vi "MFL_Check_Queue.vi"(0 "queue":refnum<queue>, 2 "error in (no error)":errorcluster) -> (3 "MFL_Monitor":T1 {"Osc 3 Freq" min=0.0 max=510000.0 format="%#_11g"; "Osc 2 Freq" min=0.0 max=510000.0 format="%#_11g"; "Osc 1 Freq" min=0.0 max=510000.0 format="%#_11g"; "Osc 0 Freq" min=0.0 max=510000.0 format="%#_11g"; "Demod Sample out 3"."Aux In 1 (V)" format="%#_5p"; "Demod Sample out 3"."Aux In 0 (V)" format="%#_5p"; "Demod Sample out 3"."X (Vrms)" format="%#_5p"; "Demod Sample out 3"."Y (Vrms)" format="%#_5p"; "Demod Sample out 3"."Osc Phase (rad)" format="%#.3g"; "Demod Sample out 2"."Aux In 1 (V)" format="%#_5p"; "Demod Sample out 2"."Aux In 0 (V)" format="%#_5p"; "Demod Sample out 2"."X (Vrms)" format="%#_5p"; "Demod Sample out 2"."Y (Vrms)" format="%#_5p"; "Demod Sample out 2"."Osc Phase (rad)" format="%#.3g"; "Demod Sample out 1"."Aux In 1 (V)" format="%#_5p"; "Demod Sample out 1"."Aux In 0 (V)" format="%#_5p"; "Demod Sample out 1"."X (Vrms)" format="%#_5p"; "Demod Sample out 1"."Y (Vrms)" format="%#_5p"; "Demod Sample out 1"."Osc Phase (rad)" format="%#.3g"; "Demod Sample out 0"."Aux In 1 (V)" format="%#_5p"; "Demod Sample out 0"."Aux In 0 (V)" format="%#_5p"; "Demod Sample out 0"."X (Vrms)" format="%#_5p"; "Demod Sample out 0"."Y (Vrms)" format="%#_5p"; "Demod Sample out 0"."Osc Phase (rad)" format="%#.3g"}, 4 "New Entries?":bool, 6 "error out":errorcluster)   [LabVIEW 2019]
uses:
  zurich_lock_in/MFLIMonitor_Cluster.ctl
  Equipment/Zurich Instruments LabOne/Public/Data/ziTypeDemodSampleEx.ctl
  Equipment/Zurich Instruments LabOne/Zurich Instruments LabOne.lvlib
panel:
  out "# elements in queue":i32
  # "Oscillators"
  # "Output Amplitudes"
  # "Frequency (Hz)"
  # "Ampl (Vpk)"
  # "0"
  # "0"
  # "1"
  # "1"
  # "2"
  # "2"
  # "3"
  # "3"
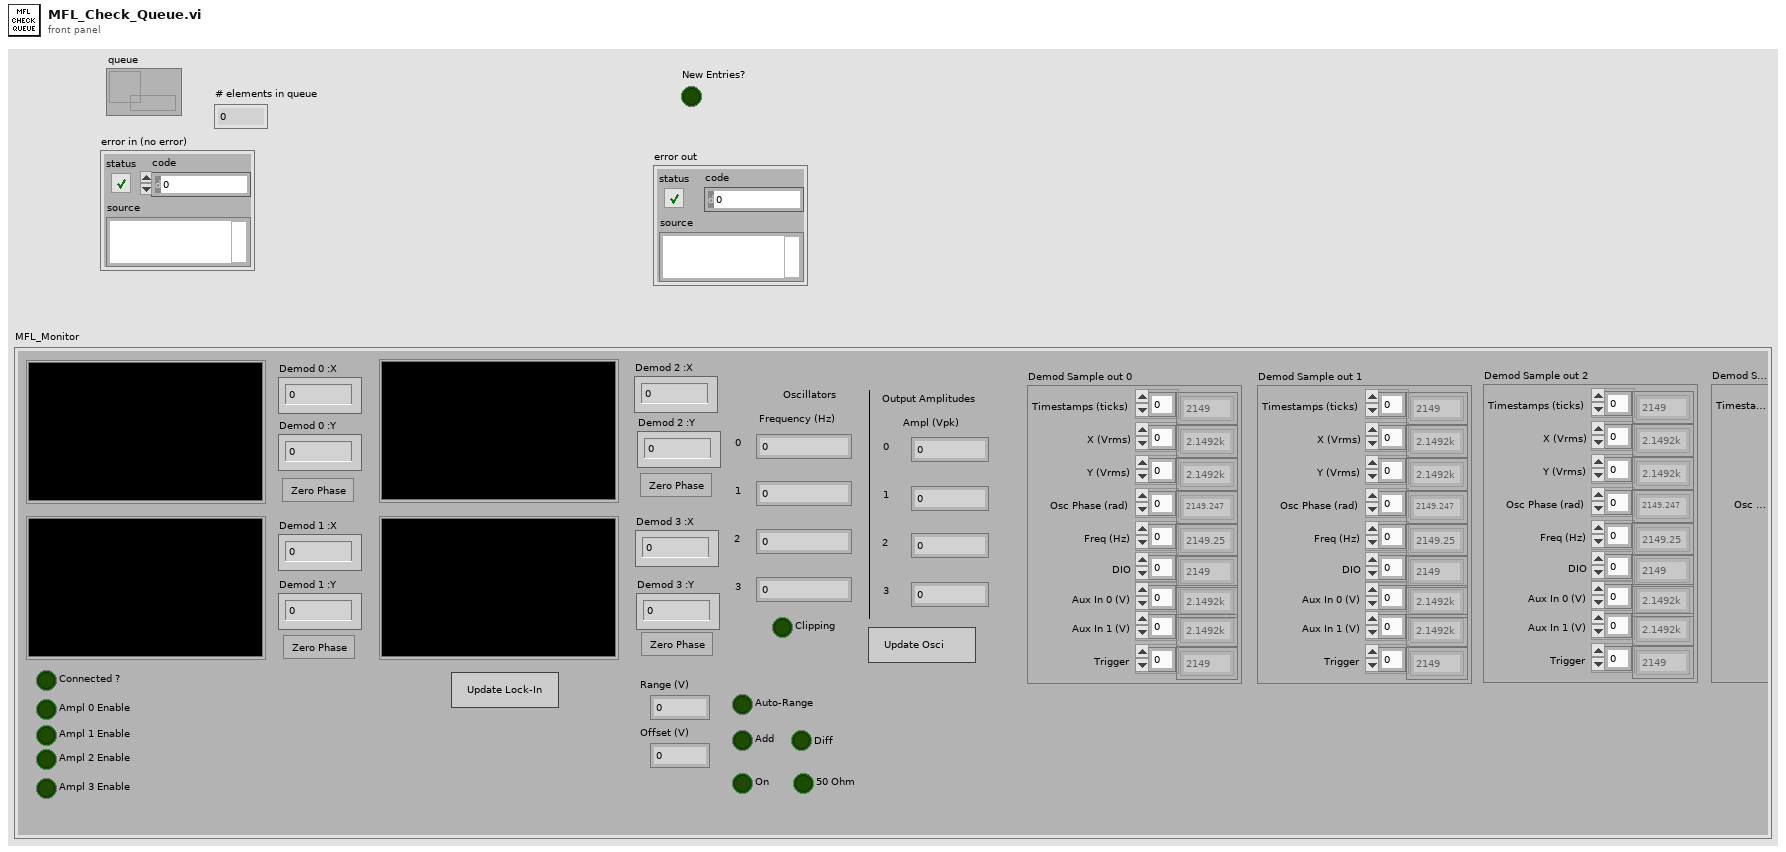
[diagram p1: front panel]
types:
  T1 = typedef "MFLIMonitor_Cluster.ctl" = cluster{"Demod 0":dbl[][], " Demod 1":dbl[][], "Demod 0 :X":dbl, "Demod 0 :Y ":dbl, "Demod 1 :X":dbl, "Demod 1 :Y ":dbl, " Demod 2":dbl[][], "Demod 3":dbl[][], "Demod 2 :X":dbl, "Demod 2 :Y ":dbl, "Demod 3 :X ":dbl, "Demod 3 :Y ":dbl, "Demod Sample out 0 ":T2, "Demod Sample out 1":T2, "Demod Sample out 2":T2, "Demod Sample out 3":T2, "Update Lock-In":bool, "Connected ?":bool, "Demod 0 Zero Phase":bool, "Demod 1 Zero Phase":bool, "Demod 2 Zero Phase":bool, "Demod 3 Zero Phase":bool, "Osc 0 Freq":dbl, "Osc 1 Freq":dbl, "Osc 2 Freq":dbl, "Osc 3 Freq":dbl, "Clipping":bool, "Range (V)":dbl, "Offset (V)":dbl, "Auto-Range":bool, "Add":bool, "Diff":bool, "On":bool, "50 Ohm":bool, "Ampl 0 Enable":bool, "Ampl 1 Enable":bool, "Ampl 2 Enable":bool, "Ampl 3 Enable":bool, "Ampl 0":dbl, "Ampl 1":dbl, "Ampl 2":dbl, "Ampl 3":dbl, "Update Osci":bool}
  T2 = typedef "Zurich Instruments LabOne.lvlib/ziTypeDemodSampleEx.ctl" = cluster{"Timestamps (ticks)":u64[], "X (Vrms)":dbl[], "Y (Vrms)":dbl[], "Osc Phase (rad)":dbl[], "Freq (Hz)":dbl[], "DIO":u32[], "Aux In 0 (V)":dbl[], "Aux In 1 (V)":dbl[], "Trigger":u32[]}
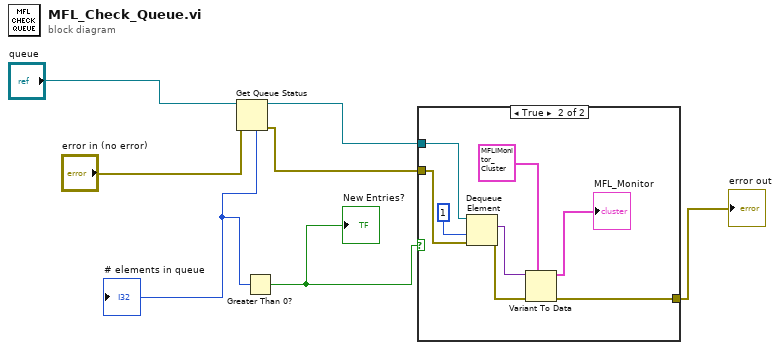
[diagram p0: block diagram]
diagram:
  n1 = Get Queue Status(queue="queue", error in (no error)="error in (no error)") -> (queue out=w3:refnum<queue>, error out=w5:errorcluster, # elements in queue=w6:i32)  [unwired: 1 in, 5 out]
  "# elements in queue" <- w6
  n2 = Greater Than 0?(x=w6) -> (x > 0?=w4:bool)
  "New Entries?" <- w4
  n3 = case shown="True" w4 {
    tunnel: w5 -> [w8 w14]
    tunnel: w3 -> [_ w16]
    tunnel: [w8 w11] -> w1
    frame False {
    }
    frame True {
      n4 = Dequeue Element(queue=w16, timeout in ms (-1)=1, error in (no error)=w14) -> (element=w13:variant, error out=w12:errorcluster)  [unwired: 2 out]
      n5 = Variant To Data(error in=w12, type=T1 {"Demod 0"=[], " Demod 1"=[], "Demod 0 :X"=0.0, "Demod 0 :Y "=0.0, "Demod 1 :X"=0.0, "Demod 1 :Y "=0.0, " Demod 2"=[], "Demod 3"=[], "Demod 2 :X"=0.0, "Demod 2 :Y "=0.0, "Demod 3 :X "=0.0, "Demod 3 :Y "=0.0, "Demod Sample out 0 "={"Timestamps (ticks)"=[], "X (Vrms)"=[], "Y (Vrms)"=[], "Osc Phase (rad)"=[], "Freq (Hz)"=[], "DIO"=[], "Aux In 0 (V)"=[], "Aux In 1 (V)"=[], "Trigger"=[]}, "Demod Sample out 1"={"Timestamps (ticks)"=[], "X (Vrms)"=[], "Y (Vrms)"=[], "Osc Phase (rad)"=[], "Freq (Hz)"=[], "DIO"=[], "Aux In 0 (V)"=[], "Aux In 1 (V)"=[], "Trigger"=[]}, "Demod Sample out 2"={"Timestamps (ticks)"=[], "X (Vrms)"=[], "Y (Vrms)"=[], "Osc Phase (rad)"=[], "Freq (Hz)"=[], "DIO"=[], "Aux In 0 (V)"=[], "Aux In 1 (V)"=[], "Trigger"=[]}, "Demod Sample out 3"={"Timestamps (ticks)"=[], "X (Vrms)"=[], "Y (Vrms)"=[], "Osc Phase (rad)"=[], "Freq (Hz)"=[], "DIO"=[], "Aux In 0 (V)"=[], "Aux In 1 (V)"=[], "Trigger"=[]}, "Update Lock-In"=FALSE, "Connected ?"=FALSE, "Demod 0 Zero Phase"=FALSE, "Demod 1 Zero Phase"=FALSE, "Demod 2 Zero Phase"=FALSE, "Demod 3 Zero Phase"=FALSE, "Osc 0 Freq"=0.0, "Osc 1 Freq"=0.0, "Osc 2 Freq"=0.0, "Osc 3 Freq"=0.0, "Clipping"=FALSE, "Range (V)"=0.0, "Offset (V)"=0.0, "Auto-Range"=FALSE, "Add"=FALSE, "Diff"=FALSE, "On"=FALSE, "50 Ohm"=FALSE, "Ampl 0 Enable"=FALSE, "Ampl 1 Enable"=FALSE, "Ampl 2 Enable"=FALSE, "Ampl 3 Enable"=FALSE, "Ampl 0"=0.0, "Ampl 1"=0.0, "Ampl 2"=0.0, "Ampl 3"=0.0, "Update Osci"=FALSE} ("MFL_Monitor"), Variant=w13) -> (data=→"MFL_Monitor":T1, error out=w11:errorcluster)
    }
  }
  "error out" <- w1
